vi "热敏电阻多通道数据采集.vi"() -> ()   [LabVIEW 2015]
uses:
  <vilib>/Utility/miscctls.llb/LVRowAndColumnTypeDef.ctl
  <vilib>/addons/_office/_exclsub.llb/font.ctl
  <vilib>/addons/_office/excel.llb/Excel Easy Table (str).vi
  <vilib>/Utility/NIReport.llb/NI_report.lvclass
  Keithley 27XX/Keithley 27XX.lvlib
  <vilib>/addons/_office/NI_ReportGenerationToolkit.lvlib
panel:
  out "消息":string
  in  "Quit":bool
  out "采集使能":bool
  in  "数据显示":string[][](table)
  in  "tab":enum32{"总线检查", "配置", "数据显示"}(tab)
  in  "Keithley2750":refnum<visa-resource-name>="COM3"
  in  "总线检查":bool
  in  "温度设置":bool
  in  "编号设置":bool
  in  "清空表格":bool
  in  "暂停":bool
  in  "采集温度":bool
  in  "目标温度":string(combo)
  in  "实测温度":string
  in  "生成报告":bool
  out "通道号":i32
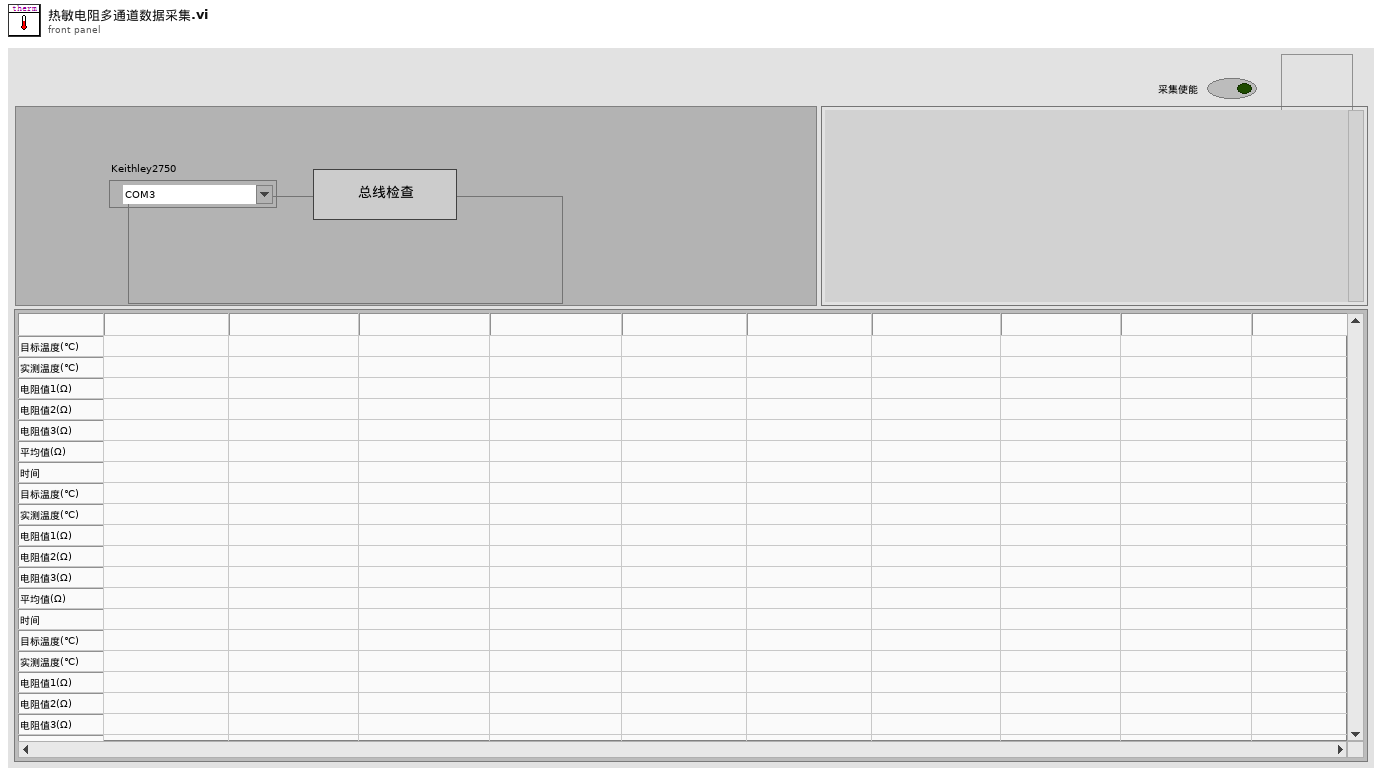
[diagram p1: front panel]
types:
  T1 = typedef "LVRowAndColumnTypeDef.ctl" = cluster{"Row":i32, "Column":i32}
  T2 = enum8{"Enabled", "Disabled", "Disabled and Grayed Out"}
  T3 = cluster{"Baud Rate (9600)":u32, "Flow Control (1: XON/XOFF)":u16, "Termination Char (0:CR)":u16}
  T4 = enum16{"maximized", "minimized", "normal", "no change"}
  T5 = enum16{"Standard Report", "HTML", "Word", "Excel"}
  T6 = typedef "NI_ReportGenerationToolkit.lvlib/font.ctl" = cluster{"font name":string, "font size":dbl, "bold":u16, "italic":u16, "underline":u16, "strike through":u16, "font color":u32}
  T7 = typedef "LVPoint32TypeDef.ctl" = cluster{"Horizontal":i32, "Vertical":i32}
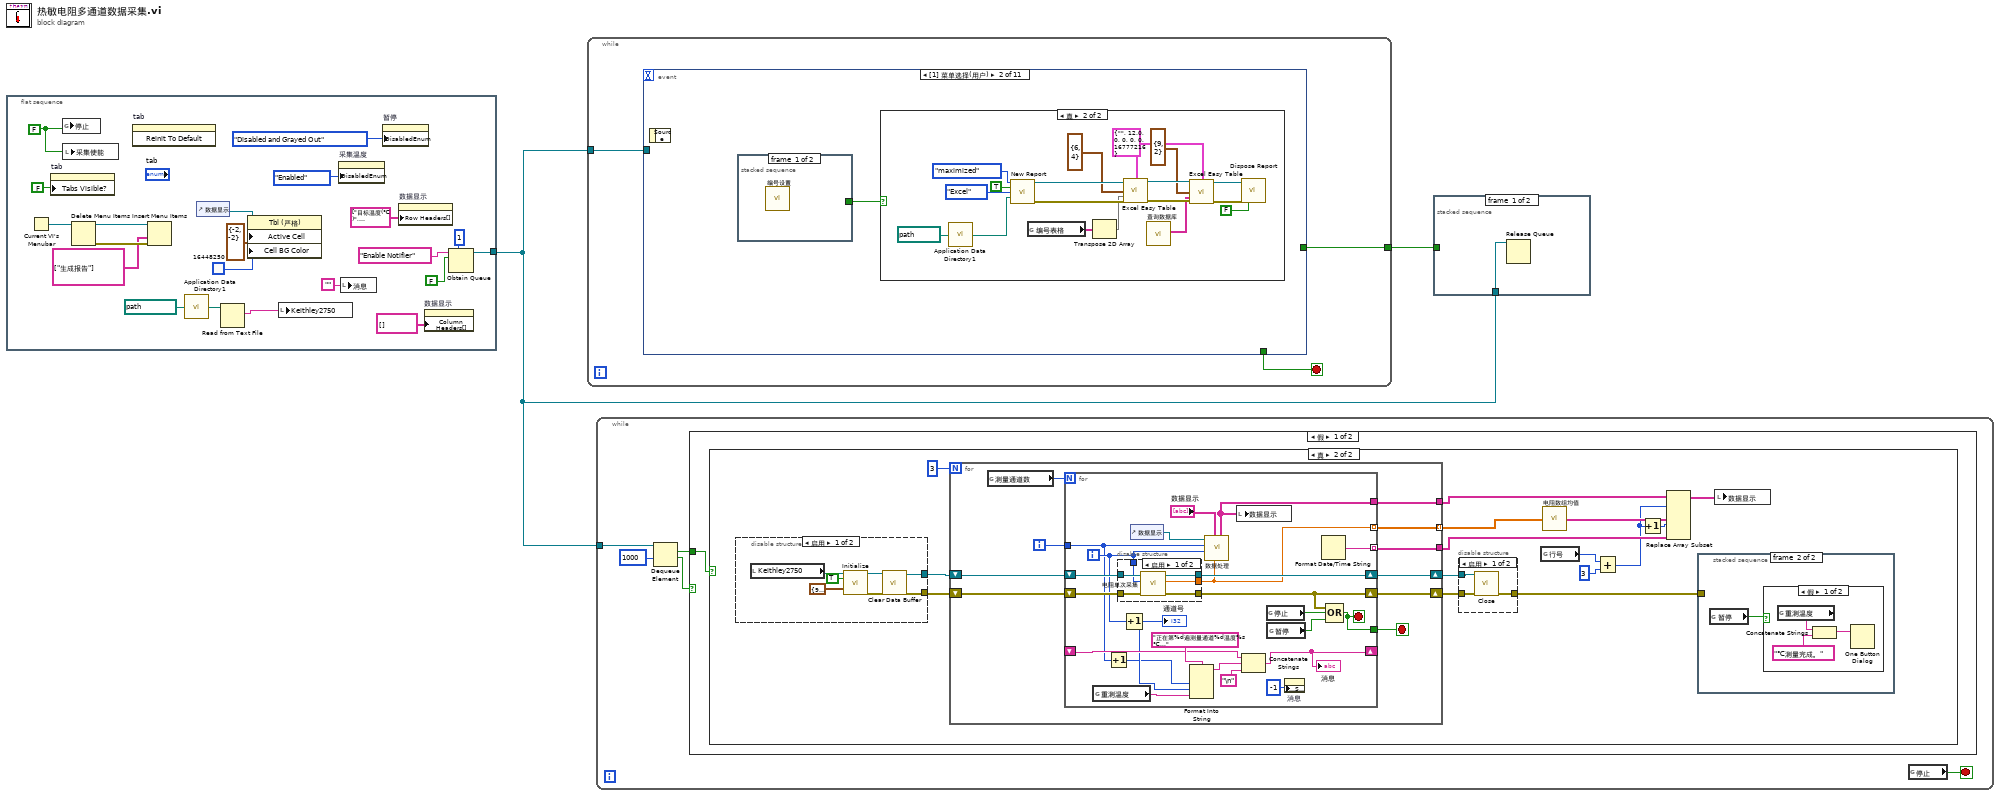
[diagram p0: block diagram]
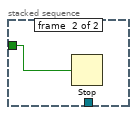
[diagram p2: hidden frame]
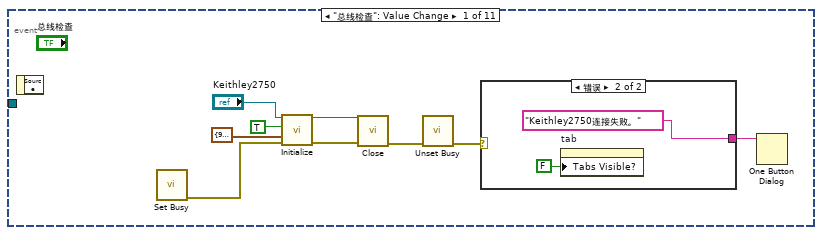
[diagram p3: hidden frame]
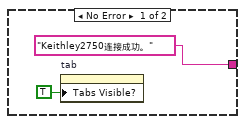
[diagram p4: hidden frame]
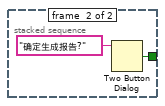
[diagram p5: hidden frame]
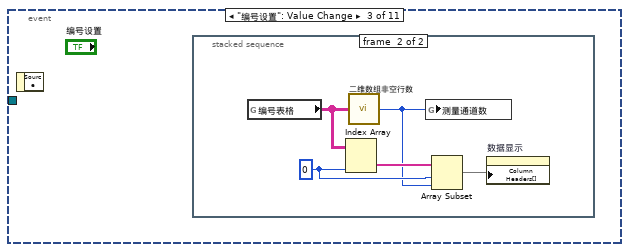
[diagram p7: hidden frame]
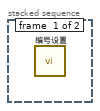
[diagram p8: hidden frame]
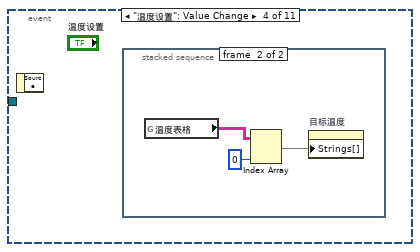
[diagram p9: hidden frame]
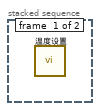
[diagram p10: hidden frame]
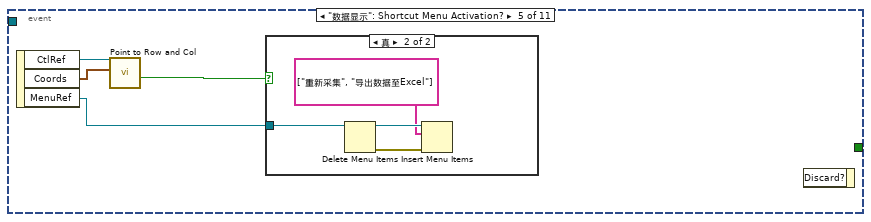
[diagram p11: hidden frame]
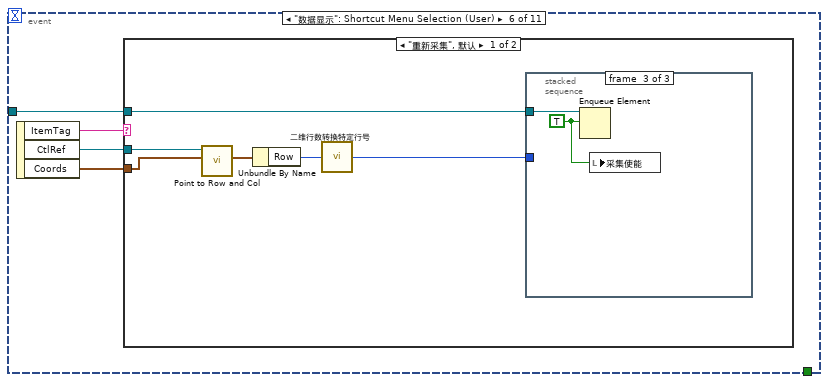
[diagram p13: hidden frame]
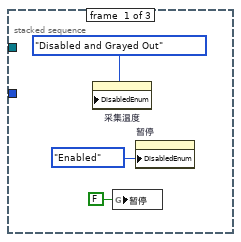
[diagram p14: hidden frame]
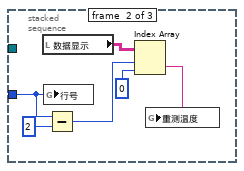
[diagram p15: hidden frame]
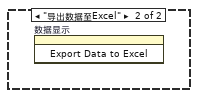
[diagram p16: hidden frame]
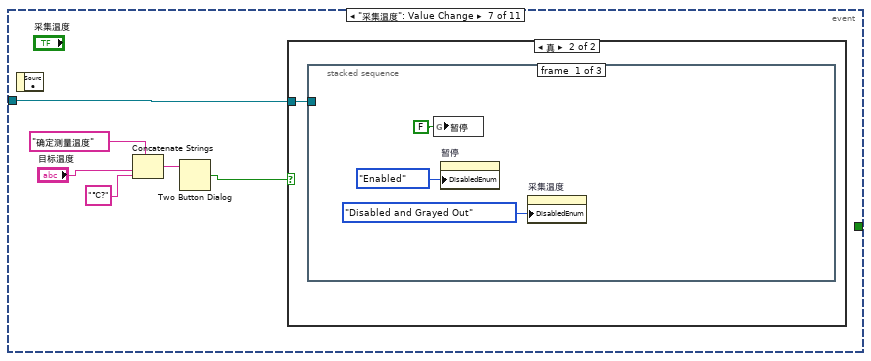
[diagram p17: hidden frame]
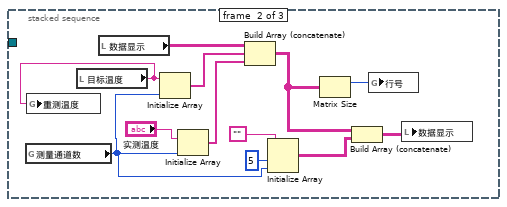
[diagram p19: hidden frame]
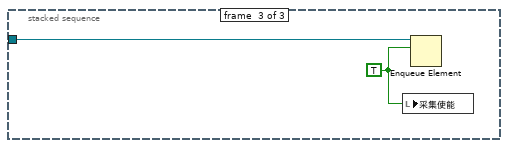
[diagram p20: hidden frame]
diagram:
  n1 = flat-sequence {
    tunnel: [w9] -> w1
    frame #0 {
      w17 = FALSE ("Excel已打开")
      n2 = Current VI's Menubar() -> (w15:refnum<k9>)
      n3 = property on="tab" class="TabCtl (严格)"("Tabs Visible?"=FALSE ("选项卡可见？")) -> ()  [unwired: 2 in, 2 out]
      n4 = global write "全局.vi" "停止"(w17) -> ()
      n5 = local write "采集使能"(w17) -> ()
      n6 = Delete Menu Items(9:w15) -> (0:w16:errorcluster, 3:w14:refnum<k9>)  [unwired: 3 in]
      n7 = invoke on="tab" class="TabCtl (严格)" method="Reinit To Default"() -> ()  [unwired: 3 in, 3 out]
      n8 = Insert Menu Items(6:w16, 7:string[] ["生成报告"] ("L10n_item tags 1"), 9:w14) -> ()  [unwired: 3 in, 3 out]
      n9 = call "Application Data Directory1.vi"("Relative path (.)"=path "串口号.txt") -> ("Application Directory (+ Relative)"=w6:path)
      n10 = control-ref of="数据显示"() -> (w20:refnum<vi>)
      n11 = Read from Text File(file (use dialog)=w6) -> (text=w5:string)  [unwired: 3 in, 3 out]
      n12 = property class="Tbl (严格)"(reference=w20, "Active Cell"=T1 {"Row"=-2, "Column"=-2} ("活动单元格:活动单元格"), "Cell BG Color"=u32 16448250 ("Origin BK Color")) -> ()  [unwired: 1 in, 2 out]
      n13 = local write "Keithley2750"(w5) -> ()
      n14 = property on="采集温度" class="Bool"("DisabledEnum"=T2."Enabled" ("禁用")) -> ()  [unwired: 2 in, 2 out]
      n15 = local write "消息"("") -> ()
      n16 = property on="暂停" class="Bool"("DisabledEnum"=T2."Disabled and Grayed Out" ("禁用")) -> ()  [unwired: 2 in, 2 out]
      n17 = property on="数据显示" class="Tbl (严格)"("Row Headers[]"=string[] ["目标温度(℃)", "实测温度(℃)", "电阻值1(Ω)", "电阻值2(Ω)", "电阻值3(Ω)", "平均值(Ω)", "时间", "目标温度(℃)", "实测温度(℃)", "电阻值1(Ω)", "电阻值2(Ω)", "电阻值3(Ω)", "平均值(Ω)", "时间", "目标温度(℃)", "实测温度(℃)", "电阻值1(Ω)", "电阻值2(Ω)", "电阻值3(Ω)", "平均值(Ω)", "时间", "目标温度(℃)", "实测温度(℃)", "电阻值1(Ω)", "电阻值2(Ω)", "电阻值3(Ω)", "平均值(Ω)", "时间", "目标温度(℃)", "实测温度(℃)", "电阻值1(Ω)", "电阻值2(Ω)", "电阻值3(Ω)", "平均值(Ω)", "时间", "目标温度(℃)", "实测温度(℃)", "电阻值1(Ω)", "电阻值2(Ω)", "电阻值3(Ω)", "平均值(Ω)", "时间", "目标温度(℃)", "实测温度(℃)", "电阻值1(Ω)", "电阻值2(Ω)", "电阻值3(Ω)", "平均值(Ω)", "时间", "目标温度(℃)", "实测温度(℃)", "电阻值1(Ω)", "电阻值2(Ω)", "电阻值3(Ω)", "平均值(Ω)", "时间", "目标温度(℃)", "实测温度(℃)", "电阻值1(Ω)", "电阻值2(Ω)", "电阻值3(Ω)", "平均值(Ω)", "时间", "目标温度(℃)", "实测温度(℃)", "电阻值1(Ω)", "电阻值2(Ω)", "电阻值3(Ω)", "平均值(Ω)", "时间", "目标温度(℃)", "实测温度(℃)", "电阻值1(Ω)", "电阻值2(Ω)", "电阻值3(Ω)", "平均值(Ω)", "时间", "目标温度(℃)", "实测温度(℃)", "电阻值1(Ω)", "电阻值2(Ω)", "电阻值3(Ω)", "平均值(Ω)", "时间", "目标温度(℃)", "实测温度(℃)", "电阻值1(Ω)", "电阻值2(Ω)", "电阻值3(Ω)", "平均值(Ω)", "时间", "目标温度(℃)", "实测温度(℃)", "电阻值1(Ω)", "电阻值2(Ω)", "电阻值3(Ω)", "平均值(Ω)", "时间", "目标温度(℃)", "实测温度(℃)", "电阻值1(Ω)", "电阻值2(Ω)", "电阻值3(Ω)", "平均值(Ω)", "时间", "目标温度(℃)", "实测温度(℃)", "电阻值1(Ω)", "电阻值2(Ω)", "电阻值3(Ω)", "平均值(Ω)", "时间", "目标温度(℃)", "实测温度(℃)", "电阻值1(Ω)", "电阻值2(Ω)", "电阻值3(Ω)", "平均值(Ω)", "时间", "目标温度(℃)", "实测温度(℃)", "电阻值1(Ω)", "电阻值2(Ω)", "电阻值3(Ω)", "平均值(Ω)", "时间", "目标温度(℃)", "实测温度(℃)", "电阻值1(Ω)", "电阻值2(Ω)", "电阻值3(Ω)", "平均值(Ω)", "时间", "目标温度(℃)", "实测温度(℃)", "电阻值1(Ω)", "电阻值2(Ω)", "电阻值3(Ω)", "平均值(Ω)", "时间", "目标温度(℃)", "实测温度(℃)", "电阻值1(Ω)", "电阻值2(Ω)", "电阻值3(Ω)", "平均值(Ω)", "时间", "目标温度(℃)", "实测温度(℃)", "电阻值1(Ω)", "电阻值2(Ω)", "电阻值3(Ω)", "平均值(Ω)", "时间", "目标温度(℃)", "实测温度(℃)", "电阻值1(Ω)", "电阻值2(Ω)", "电阻值3(Ω)", "平均值(Ω)", "时间", "目标温度(℃)", "实测温度(℃)", "电阻值1(Ω)", "电阻值2(Ω)", "电阻值3(Ω)", "平均值(Ω)", "时间", "目标温度(℃)", "实测温度(℃)", "电阻值1(Ω)", "电阻值2(Ω)", "电阻值3(Ω)", "平均值(Ω)", "时间", "目标温度(℃)", "实测温度(℃)", "电阻值1(Ω)", "电阻值2(Ω)", "电阻值3(Ω)", "平均值(Ω)", "时间", "目标温度(℃)", "实测温度(℃)", "电阻值1(Ω)", "电阻值2(Ω)", "电阻值3(Ω)", "平均值(Ω)", "时间", "目标温度(℃)", "实测温度(℃)", "电阻值1(Ω)", "电阻值2(Ω)", "电阻值3(Ω)", "平均值(Ω)", "时间", "目标温度(℃)", "实测温度(℃)", "电阻值1(Ω)", "电阻值2(Ω)", "电阻值3(Ω)", "平均值(Ω)", "时间", "目标温度(℃)", "实测温度(℃)", "电阻值1(Ω)", "电阻值2(Ω)", "电阻值3(Ω)", "平均值(Ω)", "时间", "目标温度(℃)", "实测温度(℃)", "电阻值1(Ω)", "电阻值2(Ω)", "电阻值3(Ω)", "平均值(Ω)", "时间", "目标温度(℃)", "实测温度(℃)", "电阻值1(Ω)", "电阻值2(Ω)", "电阻值3(Ω)", "平均值(Ω)", "时间", "目标温度(℃)", "实测温度(℃)", "电阻值1(Ω)", "电阻值2(Ω)", "电阻值3(Ω)", "平均值(Ω)", "时间", "目标温度(℃)", "实测温度(℃)", "电阻值1(Ω)", "电阻值2(Ω)", "电阻值3(Ω)", "平均值(Ω)", "时间", "目标温度(℃)", "实测温度(℃)", "电阻值1(Ω)", "电阻值2(Ω)", "电阻值3(Ω)", "平均值(Ω)", "时间", "目标温度(℃)", "实测温度(℃)", "电阻值1(Ω)", "电阻值2(Ω)", "电阻值3(Ω)", "平均值(Ω)", "时间", "目标温度(℃)", "实测温度(℃)", "电阻值1(Ω)", "电阻值2(Ω)", "电阻值3(Ω)", "平均值(Ω)", "时间", "目标温度(℃)", "实测温度(℃)", "电阻值1(Ω)", "电阻值2(Ω)", "电阻值3(Ω)", "平均值(Ω)", "时间", "目标温度(℃)", "实测温度(℃)", "电阻值1(Ω)", "电阻值2(Ω)", "电阻值3(Ω)", "平均值(Ω)", "时间", "目标温度(℃)", "实测温度(℃)", "电阻值1(Ω)", "电阻值2(Ω)", "电阻值3(Ω)", "平均值(Ω)", "时间", "目标温度(℃)", "实测温度(℃)", "电阻值1(Ω)", "电阻值2(Ω)", "电阻值3(Ω)", "平均值(Ω)", "时间"] ("行首字符串[]")) -> ()  [unwired: 2 in, 2 out]
      n18 = property on="数据显示" class="Tbl (严格)"("Column Headers[]"=string[] [] ("列首字符串[]")) -> ()  [unwired: 2 in, 2 out]
      n19 = Obtain Queue(max queue size (-1, unlimited)=1 ("队列最大值（-1，无限）"), name (unnamed)="Enable Notifier", element data type=FALSE ("stop confirmed")) -> (queue out=w9:refnum<queue>)  [unwired: 2 in, 2 out]
    }
  }
  n20 = while {
    tunnel: [w25] -> w2
    tunnel: w1 -> [w24]
    stop <- w26 stop-if-true
    n21 = event shown="[1] 菜单选择(用户)" {
      selector: _ -> [_ _ _ _ _ _ _ _ _ _ _]
      dyn-events: _ -> [_ _ _ _ _ _ _ _ _ _ _]
      timeout: _ -> [_ _ _ _ _ _ _ _ _ _ _]
      tunnel: [_ _ _ _ _ _ _ _ _ _ w161] -> w26
      tunnel: [_ _ _ _ _ _ _ _ _ _ w161] -> w25
      tunnel: w24 -> [_ _ _ _ _ w77 w99 w122 _ _ _]
      event "总线检查": Value Change {
        n22 = event-data() -> ()  [unwired: 1 in, 1 out]
        n23 = call <vilib>:"Set Busy.vi"() -> ("error out"=w32:errorcluster)  [unwired: 10 in, 1 out]
        n24 = call "Initialize.vi"("VISA resource name"="Keithley2750", "ID Query? (T: Yes)"=TRUE, "Serial Configuration"=T3 {"Baud Rate (9600)"=9600, "Flow Control (1: XON/XOFF)"=1, "Termination Char (0:CR)"=0}, "error in (no error)"=w32) -> ("VISA resource name out"=w34:refnum<visa-resource-name>, "error out"=w33:errorcluster)  [unwired: 10 in]
        n25 = call "Close.vi"("VISA resource name"=w34, "error in (no error)"=w33) -> ("error out"=w31:errorcluster)  [unwired: 13 in]
        n26 = call <vilib>:"Unset Busy.vi"("error in (no error)"=w31) -> ("error out"=w30:errorcluster)  [unwired: 10 in]
        n27 = case shown="错误" w30 {
          tunnel: ["Keithley2750连接成功。" ("消息") "Keithley2750连接失败。" ("消息")] -> w29
          frame No Error {
            n28 = property on="tab" class="TabCtl (严格)"("Tabs Visible?"=TRUE ("选项卡可见？")) -> ()  [unwired: 2 in, 2 out]
          }
          frame Error {
            n29 = property on="tab" class="TabCtl (严格)"("Tabs Visible?"=FALSE ("选项卡可见？")) -> ()  [unwired: 2 in, 2 out]
          }
        }
        n30 = One Button Dialog(message=w29) -> ()  [unwired: 1 in, 1 out]
      }
      event Menu Selection (User) {
        n31 = event-data() -> ()  [unwired: 1 in, 1 out]
        n32 = stacked-sequence {
          tunnel: [_ w41] -> w40
          frame #0 {
            n33 = call "编号设置.vi"() -> ()  [unwired: 12 in]
          }
          frame #1 {
            n34 = Two Button Dialog(message="确定生成报告?" ("消息")) -> (T button?=w41:bool)  [unwired: 2 in]
          }
        }
        n35 = case shown="真" w40 {
          frame False {
          }
          frame True {
            w45 = T6 {"font name"="", "font size"=12.0, "bold"=0, "italic"=0, "underline"=0, "strike through"=0, "font color"=16777216} ("font")
            n36 = call "Application Data Directory1.vi"("Relative path (.)"=path "模板.xls") -> ("Application Directory (+ Relative)"=w43:path)
            n37 = call <vilib>:"New Report.vi"("window state (normal)"=T4."maximized", "display alerts? (F)"=TRUE, "report type"=T5."Excel", "template (empty)"=w43) -> ("report out"=w55:refnum<class "NI_report.lvclass">, "error out"=w56:errorcluster)  [unwired: 10 in]
            n38 = global read "全局.vi" "编号表格"() -> (w54:string[][])
            n39 = Transpose 2D Array(2D array=w54) -> (transposed array=w52:string[][])
            n40 = call-poly <vilib>:"Excel Easy Table.vi"("report in"=w55, "font"=w45, "start (0, 0)"=cluster{"row":i32, "column":i32} {"row"=6, "column"=4}, "text data"=w52, "error in (no error)"=w56) -> ("report out"=w51:refnum<class "NI_report.lvclass">, "error out"=w50:errorcluster)  [unwired: 6 in, 3 out]
            n41 = call "查询数据库.vi"() -> ("数据"=w46:string[][])  [unwired: 11 in]
            n42 = call-poly <vilib>:"Excel Easy Table.vi"("report in"=w51, "font"=w45, "start (0, 0)"=cluster{"row":i32, "column":i32} {"row"=9, "column"=2}, "text data"=w46, "error in (no error)"=w50) -> ("report out"=w49:refnum<class "NI_report.lvclass">, "error out"=w48:errorcluster)  [unwired: 6 in, 3 out]
            n43 = call-dynamic "Dispose Report.vi"("report in"=w49, "error in (no error)"=w48, "close report? (T)"=FALSE) -> ()  [unwired: 12 in, 1 out]
          }
        }
      }
      event "编号设置": Value Change {
        n44 = event-data() -> ()  [unwired: 1 in, 1 out]
        n45 = stacked-sequence {
          frame #0 {
            n46 = call "编号设置.vi"() -> ()  [unwired: 12 in]
          }
          frame #1 {
            w63 = 0 ("禁用的索引 (列)")
            n47 = global read "全局.vi" "编号表格"() -> (w65:string[][])
            n48 = Index Array(array=w65, index (col)=w63) -> (element=w64:string[])  [unwired: 1 in]
            n49 = call "二维数组非空行数.vi"("数组"=w65) -> ("行数"=w62:i32)
            n50 = global write "全局.vi" "测量通道数"(w62) -> ()
            n51 = Array Subset(array=w64, index=w63, length=w62) -> (w61:string[])
            n52 = property on="数据显示" class="Tbl (严格)"("Column Headers[]"=w61) -> ()  [unwired: 2 in, 2 out]
          }
        }
      }
      event "温度设置": Value Change {
        n53 = event-data() -> ()  [unwired: 1 in, 1 out]
        n54 = stacked-sequence {
          frame #0 {
            n55 = call "温度设置.vi"() -> ()  [unwired: 12 in]
          }
          frame #1 {
            n56 = global read "全局.vi" "温度表格"() -> (w66:string[][])
            n57 = Index Array(array=w66, index (col)=0 ("禁用的索引 (列)")) -> (element=w68:string[])  [unwired: 1 in]
            n58 = property on="目标温度" class="CmbBox"("Strings[]"=w68) -> ()  [unwired: 2 in, 2 out]
          }
        }
      }
      event "数据显示": Shortcut Menu Activation? {
        n59 = event-data() -> ("CtlRef"=w71:refnum<vi>, "Coords"=w72:T7, "MenuRef"=w69:refnum<k9>)  [unwired: 1 in]
        n60 = call "Point to Row and Col.vi"("点"=w72, "Table Ref In"=w71) -> ("边界内？"=w70:bool)  [unwired: 6 in, 3 out]
        n61 = case shown="真" w70 {
          tunnel: w69 -> [_ w74]
          frame False {
          }
          frame True {
            n62 = Delete Menu Items(9:w74) -> (0:w76:errorcluster, 3:w75:refnum<k9>)  [unwired: 3 in]
            n63 = Insert Menu Items(6:w76, 8:string[] ["重新采集", "导出数据至Excel"] ("项名称"), 9:w75) -> ()  [unwired: 3 in, 3 out]
          }
        }
        n64 = event-data() -> ()  [unwired: 2 in, 1 out]
      }
      event "数据显示": Shortcut Menu Selection (User) {
        n65 = event-data() -> ("ItemTag"=w80:string, "CtlRef"=w78:refnum<vi>, "Coords"=w79:T7)  [unwired: 1 in]
        n66 = case shown="\"重新采集\", 默认" w80 {
          tunnel: w79 -> [w85 _]
          tunnel: w78 -> [w86 _]
          tunnel: w77 -> [w82 _]
          frame "重新采集", Default {
            n67 = call "Point to Row and Col.vi"("点"=w85, "Table Ref In"=w86) -> ("单元格位置"=w84:T1)  [unwired: 6 in, 3 out]
            n68 = Unbundle By Name(w84) -> ("Row"=w83:i32)
            n69 = call "二维行数转换特定行号.vi"("行数"=w83) -> ("目标温度行号"=w81:i32)
            n70 = stacked-sequence {
              tunnel: w82 -> [_ _ w96]
              tunnel: w81 -> [_ w95 _]
              frame #0 {
                n71 = property on="采集温度" class="Bool"("DisabledEnum"=T2."Disabled and Grayed Out" ("禁用")) -> ()  [unwired: 2 in, 2 out]
                n72 = global write "全局.vi" "暂停"(FALSE ("暂停")) -> ()
                n73 = property on="暂停" class="Bool"("DisabledEnum"=T2."Enabled" ("禁用")) -> ()  [unwired: 2 in, 2 out]
              }
              frame #1 {
                n74 = local read "数据显示"() -> (w93:string[][])
                n75 = global write "全局.vi" "行号"(w95) -> ()
                n76 = Subtract(x=w95, y=2) -> (x-y=w92:i32)
                n77 = Index Array(array=w93, index (row)=w92, index (col)=0 ("禁用的索引 (列)")) -> (element=w90:string)
                n78 = global write "全局.vi" "重测温度"(w90) -> ()
              }
              frame #2 {
                w97 = TRUE ("采集使能")
                n79 = Enqueue Element(queue=w96, element=w97) -> ()  [unwired: 2 in, 3 out]
                n80 = local write "采集使能"(w97) -> ()
              }
            }
          }
          frame "导出数据至Excel" {
            n81 = invoke on="数据显示" class="Tbl (严格)" method="Export Data to Excel"() -> ()  [unwired: 3 in, 3 out]
          }
        }
      }
      event "采集温度": Value Change {
        n82 = event-data() -> ()  [unwired: 1 in, 1 out]
        n83 = Concatenate Strings("确定测量温度", "目标温度", "℃?") -> (w103:string)
        n84 = Two Button Dialog(message=w103) -> (T button?=w100:bool)  [unwired: 2 in]
        n85 = case shown="真" w100 {
          tunnel: w99 -> [_ w104]
          frame False {
          }
          frame True {
            n86 = stacked-sequence {
              tunnel: w104 -> [_ _ w120]
              frame #0 {
                n87 = global write "全局.vi" "暂停"(FALSE ("暂停")) -> ()
                n88 = property on="暂停" class="Bool"("DisabledEnum"=T2."Enabled" ("禁用")) -> ()  [unwired: 2 in, 2 out]
                n89 = property on="采集温度" class="Bool"("DisabledEnum"=T2."Disabled and Grayed Out" ("禁用")) -> ()  [unwired: 2 in, 2 out]
              }
              frame #1 {
                n90 = global read "全局.vi" "测量通道数"() -> (w110:i32)
                n91 = local read "目标温度"() -> (w108:string)
                n92 = global write "全局.vi" "重测温度"(w108) -> ()
                n93 = local read "数据显示"() -> (w115:string[][])
                n94 = Initialize Array(w108, w110) -> (w119:string[])
                n95 = Initialize Array("实测温度", w110) -> (w118:string[])
                n96 = Build Array (concatenate)(w115, w119, w118) -> (w113:string[][])
                n97 = Initialize Array("", 5 ("维数大小"), w110) -> (w114:string[][])
                n98 = Matrix Size(0:w113) -> (1:w111:i32)  [unwired: 1 out]
                n99 = Build Array (concatenate)(w113, w114) -> (w112:string[][])
                n100 = global write "全局.vi" "行号"(w111) -> ()
                n101 = local write "数据显示"(w112) -> ()
              }
              frame #2 {
                w121 = TRUE ("采集使能")
                n102 = local write "采集使能"(w121) -> ()
                n103 = Enqueue Element(queue=w120, element=w121) -> ()  [unwired: 2 in, 3 out]
              }
            }
          }
        }
      }
      event "暂停": Value Change {
        n104 = event-data() -> ()  [unwired: 1 in, 1 out]
        n105 = property on="暂停" class="Bool"("DisabledEnum"=T2."Disabled and Grayed Out" ("禁用")) -> ()  [unwired: 2 in, 2 out]
        n106 = property on="采集温度" class="Bool"("DisabledEnum"=T2."Enabled" ("禁用")) -> ()  [unwired: 2 in, 2 out]
        n107 = flat-sequence {
          tunnel: [w126] -> w123
          tunnel: w122 -> [w126]
          tunnel: w123 -> [w128]
          frame #0 {
            n108 = global write "全局.vi" "暂停"(TRUE ("暂停")) -> ()
          }
          frame #1 {
            w129 = FALSE ("采集使能")
            n109 = local write "采集使能"(w129) -> ()
            n110 = Enqueue Element(queue=w128, element=w129) -> ()  [unwired: 2 in, 3 out]
          }
        }
      }
      event "清空表格": Value Change {
        n111 = event-data() -> ()  [unwired: 1 in, 1 out]
        n112 = control-ref of="数据显示"() -> (w132:refnum<vi>)
        n113 = local write "数据显示"(string[][] [] ("数据显示")) -> ()
        n114 = property class="Tbl (严格)"(reference=w132, "Active Cell"=T1 {"Row"=-2, "Column"=-2} ("活动单元格:活动单元格"), "Cell BG Color"=u32 16448250 ("Origin BK Color")) -> ()  [unwired: 1 in, 2 out]
      }
      event "生成报告": Value Change {
        n115 = event-data() -> ()  [unwired: 1 in, 1 out]
        n116 = stacked-sequence {
          frame #0 {
            n117 = call <vilib>:"Set Busy.vi"() -> ("error out"=w134:errorcluster)  [unwired: 10 in, 1 out]
            n118 = flat-sequence {
              tunnel: w134 -> [_]
              frame #0 {
                n119 = local read "消息"() -> (w140:string)
                n120 = Concatenate Strings(w140, "正在写入数据库..." ("字符串")) -> (w137:string)
                n121 = local write "消息"(w137) -> ()
                n122 = property on="消息" class="Str"("Text.Scroll Position"=-1) -> ()  [unwired: 2 in, 2 out]
              }
            }
            n123 = control-ref of="数据显示"() -> (w136:refnum<vi>)
            n124 = call "写入数据库.vi"("数据显示"=w136, "错误输入（无错误）"=w134) -> ("错误输出"=w135:errorcluster)
            n125 = call <vilib>:"Unset Busy.vi"("error in (no error)"=w135) -> ()  [unwired: 10 in, 1 out]
          }
          frame #1 {
            n126 = Two Button Dialog(message="确定生成报告?" ("消息")) -> (T button?=w141:bool)  [unwired: 2 in]
            n127 = case shown="真" w141 {
              frame False {
              }
              frame True {
                w145 = T6 {"font name"="", "font size"=12.0, "bold"=0, "italic"=0, "underline"=0, "strike through"=0, "font color"=16777216} ("font")
                n128 = call "Application Data Directory1.vi"("Relative path (.)"=path "模板.xls") -> ("Application Directory (+ Relative)"=w143:path)
                n129 = call <vilib>:"New Report.vi"("window state (normal)"=T4."maximized", "display alerts? (F)"=TRUE, "report type"=T5."Excel", "template (empty)"=w143) -> ("report out"=w155:refnum<class "NI_report.lvclass">, "error out"=w156:errorcluster)  [unwired: 10 in]
                n130 = global read "全局.vi" "编号表格"() -> (w154:string[][])
                n131 = Transpose 2D Array(2D array=w154) -> (transposed array=w152:string[][])
                n132 = call-poly <vilib>:"Excel Easy Table.vi"("report in"=w155, "font"=w145, "start (0, 0)"=cluster{"row":i32, "column":i32} {"row"=6, "column"=4}, "text data"=w152, "error in (no error)"=w156) -> ("report out"=w151:refnum<class "NI_report.lvclass">, "error out"=w150:errorcluster)  [unwired: 6 in, 3 out]
                n133 = call "查询数据库.vi"() -> ("数据"=w146:string[][])  [unwired: 11 in]
                n134 = call-poly <vilib>:"Excel Easy Table.vi"("report in"=w151, "font"=w145, "start (0, 0)"=cluster{"row":i32, "column":i32} {"row"=9, "column"=2}, "text data"=w146, "error in (no error)"=w150) -> ("report out"=w149:refnum<class "NI_report.lvclass">, "error out"=w148:errorcluster)  [unwired: 6 in, 3 out]
                n135 = call-dynamic "Dispose Report.vi"("report in"=w149, "error in (no error)"=w148, "close report? (T)"=FALSE) -> ()  [unwired: 12 in, 1 out]
              }
            }
          }
        }
      }
      event "Quit": Value Change {
        w161 = TRUE
        n136 = event-data() -> ()  [unwired: 1 in, 1 out]
        n137 = global write "全局.vi" "停止"(w161) -> ()
      }
    }
  }
  n138 = while {
    tunnel: w1 -> [w165]
    stop <- w166 stop-if-true
    n139 = Dequeue Element(queue=w165, timeout in ms (-1)=1000 ("超时毫秒(-1)")) -> (element=w162:bool, timed out?=w163:bool)  [unwired: 1 in, 2 out]
    n140 = case shown="假" w163 {
      tunnel: w162 -> [w167 _]
      frame False {
        n141 = case shown="真" w167 {
          frame False {
          }
          frame True {
            n142 = disable-structure shown="启用" {
              disable-tunnel: [w192 _] -> w181
              disable-tunnel: [w191 _] -> w180
              frame Enabled {
                n143 = local read "Keithley2750"() -> (w190:refnum<visa-resource-name>)
                n144 = call "Initialize.vi"("VISA resource name"=w190, "ID Query? (T: Yes)"=TRUE, "Serial Configuration"=T3 {"Baud Rate (9600)"=9600, "Flow Control (1: XON/XOFF)"=1, "Termination Char (0:CR)"=0}) -> ("VISA resource name out"=w188:refnum<visa-resource-name>, "error out"=w187:errorcluster)  [unwired: 11 in]
                n145 = call "Clear Data Buffer.vi"("VISA resource name"=w188, "error in (no error)"=w187) -> ("VISA resource name out"=w192:refnum<visa-resource-name>, "error out"=w191:errorcluster)  [unwired: 12 in]
              }
              frame Disabled {
              }
            }
            n146 = for {
              N: 3 -> [_]
              shift-right: [w208] -> w178
              shift-left: w180 -> [w207]
              shift-right: [w209] -> w177
              shift-left: w181 -> [w206]
              tunnel: [w203] -> w179 mode=indexing
              tunnel: [w200] -> w171
              tunnel: [w201] -> w175
              i -> [w202]
              stop <- w205 stop-if-true
              n147 = global read "全局.vi" "测量通道数"() -> (w204:i32)
              n148 = for {
                N: w204 -> [_]
                shift-right: [w229] -> w208
                shift-left: w207 -> [w232]
                shift-right: [w230] -> w209
                shift-left: w206 -> [w231]
                tunnel: [w228] -> w205
                tunnel: [w224] -> w203 mode=indexing
                tunnel: w202 -> [w212]
                tunnel: [w223] -> w201
                tunnel: [w222] -> w200 mode=indexing
                shift-right: [w214] -> _
                shift-left: _ -> [w215]
                i -> [w221]
                stop <- w228 stop-if-true
                n149 = global read "全局.vi" "重测温度"() -> (w218:string)
                n150 = Increment(x=w212) -> (x+1=w211:i32)
                n151 = disable-structure shown="启用" {
                  disable-tunnel: w232 -> [w238 _]
                  disable-tunnel: w231 -> [w237 _]
                  disable-tunnel: [w236 _] -> w230
                  disable-tunnel: [w235 _] -> w229
                  disable-tunnel: [w234 w239] -> w224
                  disable-tunnel: w221 -> [w233 _]
                  frame Enabled {
                    n152 = call "电阻单次采集.vi"("错误输入（无错误）"=w238, "通道数"=w233, "VISA引用句柄输入"=w237) -> ("错误输出"=w235:errorcluster, "测量结果"=w234:dbl, "VISA引用句柄输出"=w236:refnum<visa-resource-name>)  [unwired: 5 in, 1 out]
                  }
                  frame Disabled {
                    n153 = Random Number (0-1)() -> (number: 0 to 1=w239:dbl)
                  }
                }
                n154 = Increment(x=w221) -> (x+1=w213:i32)
                "通道号" <- w213
                n155 = control-ref of="数据显示"() -> (w225:refnum<vi>)
                n156 = Format Into String(format string="正在第%d遍测量通道%d温度%s℃...", w211, w213, w218) -> (resulting string=w216:string)  [unwired: 2 in, 1 out]
                n157 = call "数据处理.vi"("电阻值"=w224, "数据显示输入"="数据显示", "列数"=w221, "行数"=w212, "数据显示"=w225) -> ("数据显示输出"=w223:string[][])  [unwired: 6 in]
                n158 = local write "数据显示"(w223) -> ()
                n159 = Concatenate Strings(w215, w216, "\n") -> (w214:string)
                "消息" <- w214
                n160 = global read "全局.vi" "停止"() -> (w227:bool)
                n161 = global read "全局.vi" "暂停"() -> (w226:bool)
                n162 = property on="消息" class="Str"("Text.Scroll Position"=-1) -> ()  [unwired: 2 in, 2 out]
                n163 = Format Date/Time String() -> (date/time string=w222:string)  [unwired: 3 in]
                n164 = Compound Arithmetic op=OR ("复合运算")(w229, w227, w226) -> (w228:bool)
              }
            }
            n165 = disable-structure shown="启用" {
              disable-tunnel: w178 -> [w185 _]
              disable-tunnel: w177 -> [w184 _]
              disable-tunnel: [w183 _] -> w176
              frame Enabled {
                n166 = call "Close.vi"("VISA resource name"=w184, "error in (no error)"=w185) -> ("error out"=w183:errorcluster)  [unwired: 13 in]
              }
              frame Disabled {
              }
            }
            n167 = global read "全局.vi" "行号"() -> (w174:i32)
            n168 = call "电阻数组均值.vi"("电阻数组"=w179) -> ("均值"=w172:string[])
            n169 = Add(x=w174, y=3) -> (x+y=w169:i32)
            n170 = Increment(x=w169) -> (x+1=w168:i32)
            n171 = Replace Array Subset(array=w175, new element #1=w172, index (row) #1=w169, new element #2=w171, index (row) #2=w168) -> (w170:string[][])  [unwired: 2 in]
            n172 = stacked-sequence {
              tunnel: w176 -> [_ _]
              frame #0 {
                n173 = property on="采集温度" class="Bool"("DisabledEnum"=0) -> ()  [unwired: 2 in, 2 out]
                n174 = property on="暂停" class="Bool"("DisabledEnum"=2) -> ()  [unwired: 2 in, 2 out]
                "采集使能" <- FALSE ("采集使能")
              }
              frame #1 {
                n175 = global read "全局.vi" "暂停"() -> (w196:bool)
                n176 = case shown="假" w196 {
                  frame False {
                    n177 = global read "全局.vi" "重测温度"() -> (w197:string)
                    n178 = Concatenate Strings(w197, "℃测量完成。") -> (w198:string)
                    n179 = One Button Dialog(message=w198) -> ()  [unwired: 1 in, 1 out]
                  }
                  frame True {
                  }
                }
              }
            }
            n180 = local write "数据显示"(w170) -> ()
          }
        }
      }
      frame True {
      }
    }
    n181 = global read "全局.vi" "停止"() -> (w166:bool)
  }
  n182 = stacked-sequence {
    tunnel: w2 -> [_ w241]
    tunnel: w1 -> [w240 _]
    frame #0 {
      n183 = Release Queue(queue=w240) -> ()  [unwired: 2 in, 3 out]
    }
    frame #1 {
      n184 = Stop(stop? (T)=w241) -> ()
    }
  }
